vi "Case Structure Test.vi"() -> ()   [LabVIEW 2019]
uses:
  <vilib>/gpm_packages/@cs/test-executive/Source/Test Executive/TestExecutive/Test Executive.lvclass
  C:/Program Files/National Instruments/LabVIEW 2019/vi.lib/gpm_packages/@cs/test-executive/Source/Test Executive/ITestExecutive/ITest Executive.lvclass
  <vilib>/gpm_packages/@cs/run-time-assertions/Source/Assert Equal/Assert Equal.lvclass
  C:/Program Files/National Instruments/LabVIEW 2019/vi.lib/gpm_packages/@cs/run-time-assertions/Source/Assert/Assert.lvclass
  <vilib>/gpm_packages/@cs/run-time-assertions/Source/Assert Greater/Assert Greater.lvclass
  <vilib>/gpm_packages/@cs/run-time-assertions/Source/Assert Less/Assert Less.lvclass
  <vilib>/gpm_packages/@cs/test-executive/Source/Test Executive/Executioner/Executioner.lvclass
  <vilib>/gpm_packages/@cs/persistence/source/XML/XML.lvclass
  C:/Program Files/National Instruments/LabVIEW 2019/vi.lib/gpm_packages/@cs/persistence/source/IPersist/IPersist.lvclass
  e472b746-f4c1-47e9-9711-c7fa7be09181.vi
  ab0fdcf2-3a2d-4a0b-9adf-5da32de36cdd.vi
  99c89cbf-b02e-47c8-8025-58ec5524d82c.vi
  fd6ea1e6-9cba-4bab-b7d6-62b422661ca4.vi
  21af0a36-f5b0-40a4-aa97-dd1ed5091c43.vi
  9cf53736-387a-4554-ab29-2a757f105b86.vi
  bc4700c4-b3ec-42c3-ab81-83467d48079d.vi
  <vilib>/Utility/error.llb/Error Cluster From Error Code.vi
  <vilib>/gpm_packages/@cs/test-executive/Source/Test Executive/ITestExecutive/ITest Executive.lvclass
  <vilib>/gpm_packages/@cs/test-executive/Source/Test Executive/TestExecutive Ref/TestExecutive Ref.lvclass
panel:
  out "Conditional Branches In":string[](array[string])
  out "Conditional Branches out":string[](array[string])
  in  "stop 2":bool
  in  "stop":bool
  in  "Tree":string(tree)
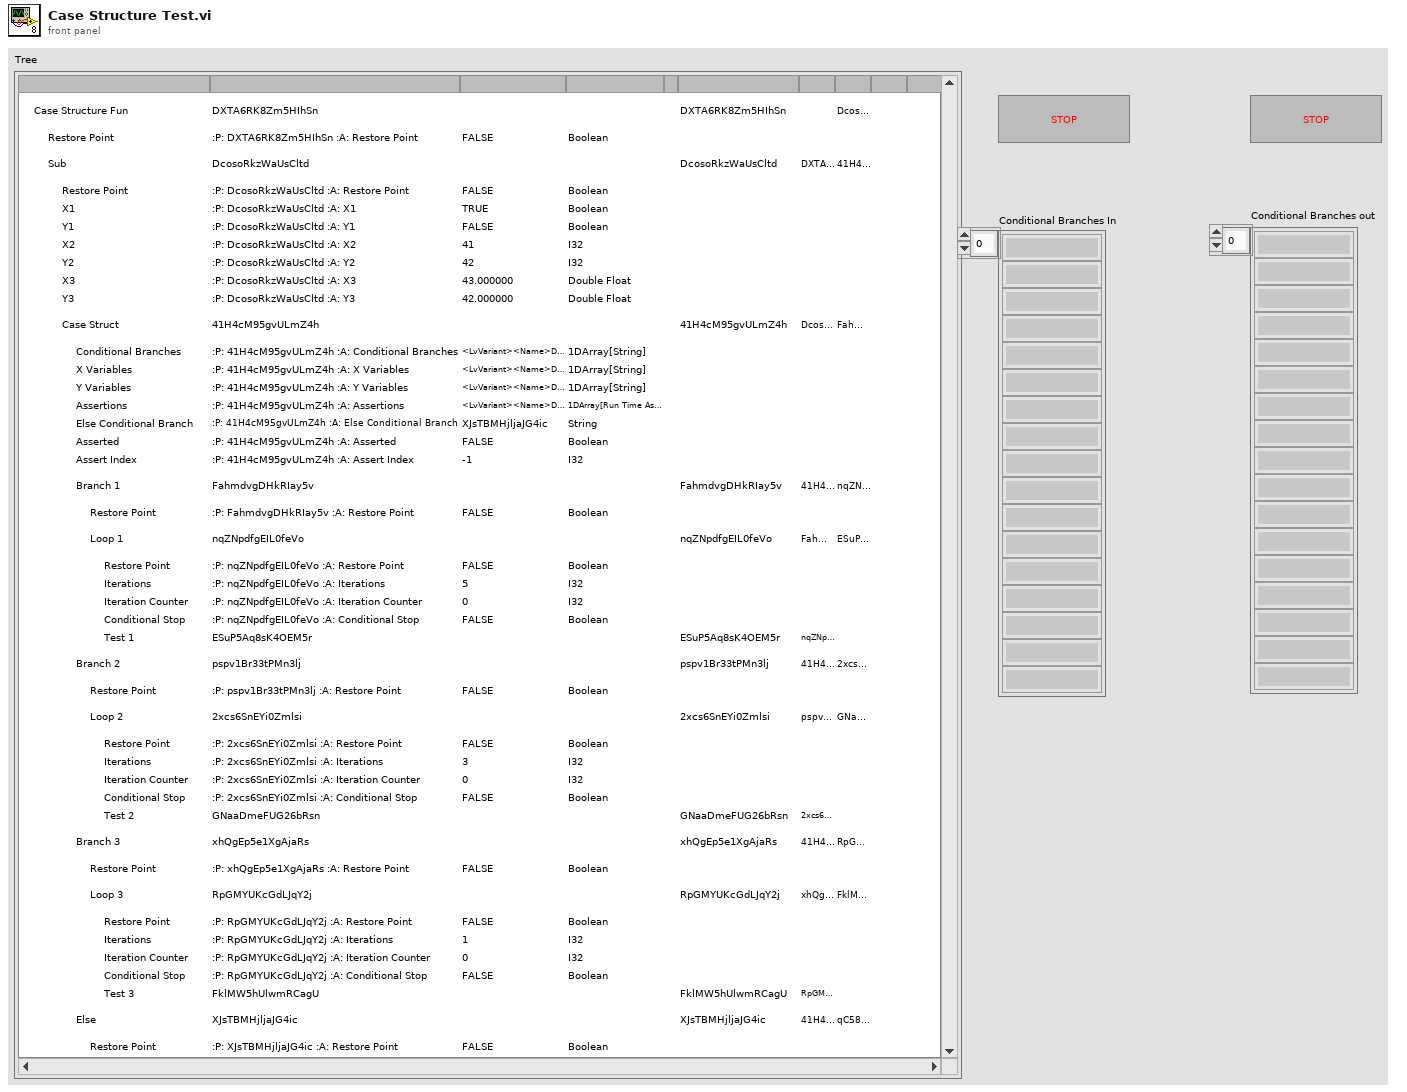
[diagram p1: front panel]
types:
  T1 = cluster{"Left Cell String":string, "Child Text":string[], "Child Tag":string, "Item Indent":i32, "Child Only?":bool, "Glyph Index":i32}[]
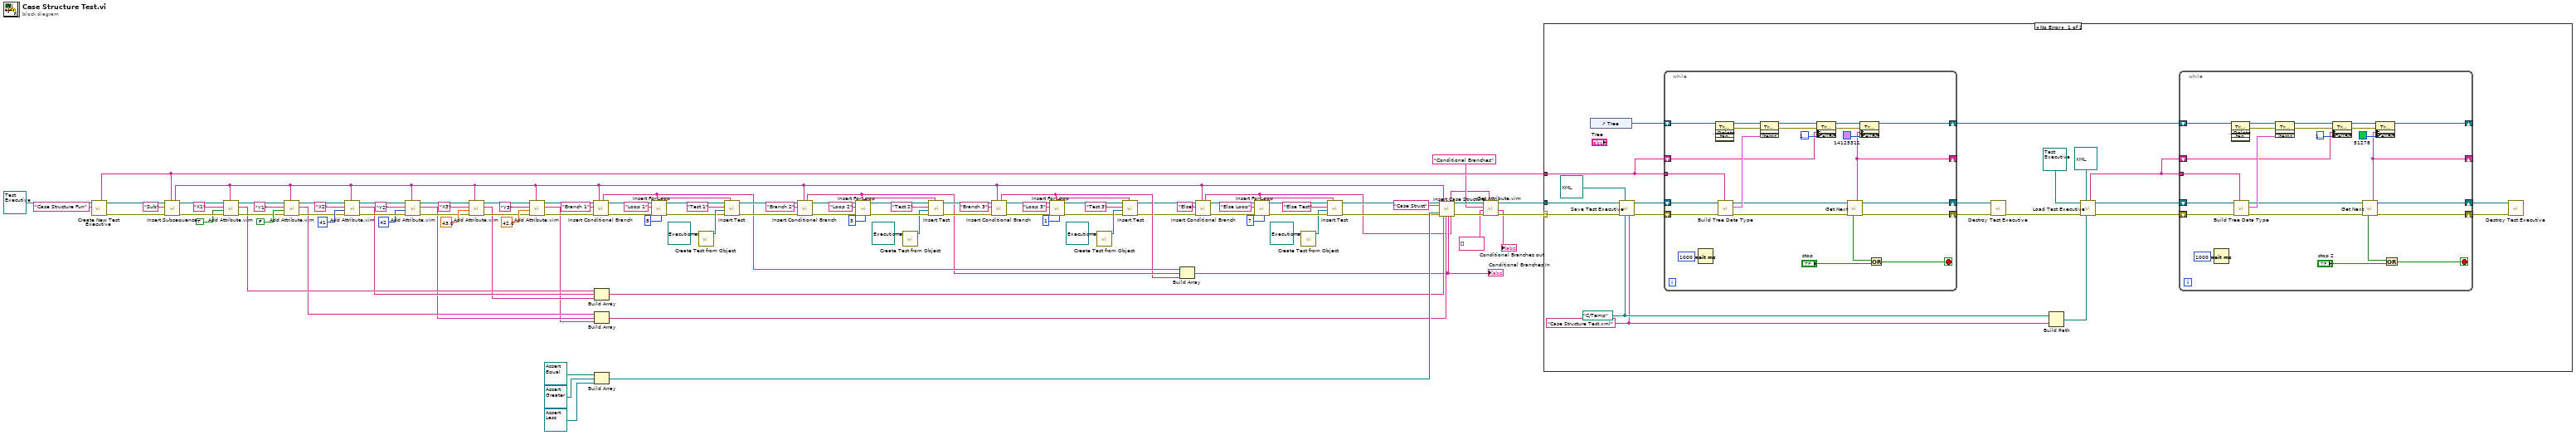
[diagram p0: block diagram]
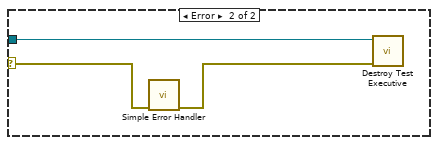
[diagram p2: hidden frame]
diagram:
  n1 = call <vilib>:"Create New Test Executive.vi"("Name"="Case Structure Fun", "Test Executive"=refnum<class "Test Executive.lvclass"> refnum ("Test Executive.lvlib:Test Executive.lvclass")) -> ("error out"=w107:errorcluster, "Test Executive Ref"=w109:refnum<data-value>, "Test Executive ID out"=w11:string)  [unwired: 7 in]
  n2 = call <vilib>:"Insert Subsequence.vi"("Parent ID"=w11, "error in (no error)"=w107, "Name"="Sub", "Test Executive Ref"=w109) -> ("error out"=w105:errorcluster, "Test Executive Ref out"=w106:refnum<data-value>, "Unique ID out"=w7:string)  [unwired: 4 in, 1 out]
  n3 = call "Add Attribute.vim"("ID"=w7, "error in (no error)"=w105, "Attribute"=TRUE, "Attribute Name"="X1", "Test Executive Ref"=w106) -> ("error out"=w99:errorcluster, "Attribute ID out"=w39:string, "Test Executive Ref out"=w100:refnum<data-value>)  [unwired: 3 in, 1 out]
  n4 = call "Add Attribute.vim"("ID"=w7, "error in (no error)"=w99, "Attribute"=FALSE, "Attribute Name"="Y1", "Test Executive Ref"=w100) -> ("error out"=w91:errorcluster, "Attribute ID out"=w36:string, "Test Executive Ref out"=w92:refnum<data-value>)  [unwired: 3 in, 1 out]
  n5 = call "Add Attribute.vim"("ID"=w7, "error in (no error)"=w91, "Attribute"=41, "Attribute Name"="X2", "Test Executive Ref"=w92) -> ("error out"=w98:errorcluster, "Attribute ID out"=w38:string, "Test Executive Ref out"=w97:refnum<data-value>)  [unwired: 3 in, 1 out]
  n6 = call "Add Attribute.vim"("ID"=w7, "error in (no error)"=w98, "Attribute"=42, "Attribute Name"="Y2", "Test Executive Ref"=w97) -> ("error out"=w83:errorcluster, "Attribute ID out"=w35:string, "Test Executive Ref out"=w84:refnum<data-value>)  [unwired: 3 in, 1 out]
  n7 = call "Add Attribute.vim"("ID"=w7, "error in (no error)"=w83, "Attribute"=43.0, "Attribute Name"="X3", "Test Executive Ref"=w84) -> ("error out"=w85:errorcluster, "Attribute ID out"=w37:string, "Test Executive Ref out"=w86:refnum<data-value>)  [unwired: 3 in, 1 out]
  n8 = call "Add Attribute.vim"("ID"=w7, "error in (no error)"=w85, "Attribute"=42.0, "Attribute Name"="Y3", "Test Executive Ref"=w86) -> ("error out"=w80:errorcluster, "Attribute ID out"=w34:string, "Test Executive Ref out"=w82:refnum<data-value>)  [unwired: 3 in, 1 out]
  n9 = call <vilib>:"Insert Conditional Branch.vi"("Parent ID"=w7, "error in (no error)"=w80, "Name"="Branch 1", "Test Executive Ref"=w82) -> ("error out"=w76:errorcluster, "Test Executive Ref out"=w78:refnum<data-value>, "Unique ID out"=w31:string)  [unwired: 4 in, 1 out]
  n10 = Build Array(w39, w38, w37) -> (w33:string[])
  n11 = Build Array(w36, w35, w34) -> (w32:string[])
  n12 = Build Array(refnum<class "Assert Equal.lvclass"> refnum ("Run Time Assertions.lvlib:Assert Equal.lvclass"), refnum<class "Assert Greater.lvclass"> refnum ("Run Time Assertions.lvlib:Assert Greater.lvclass"), refnum<class "Assert Less.lvclass"> refnum ("Run Time Assertions.lvlib:Assert Less.lvclass")) -> (w40:refnum<class "Assert.lvclass">[])
  n13 = call <vilib>:"Insert For Loop.vi"("Loop Iterations"=5, "Parent ID"=w31, "error in (no error)"=w76, "Name"="Loop 1", "Test Executive Ref"=w78) -> ("error out"=w72:errorcluster, "Test Executive Ref out"=w71:refnum<data-value>, "Unique ID out"=w70:string)  [unwired: 3 in, 1 out]
  n14 = call <vilib>:"Create Test from Object.vi"("Test"=refnum<class "Executioner.lvclass"> refnum ("Test Executive.lvlib:Executioner.lvclass")) -> ("Test"=w73:refnum<class "Executioner.lvclass">)  [unwired: 10 in]
  n15 = call <vilib>:"Insert Test.vi"("Parent ID"=w70, "error in (no error)"=w72, "Test"=w73, "Name"="Test 1", "Test Executive Ref"=w71) -> ("error out"=w57:errorcluster, "Test Executive Ref out"=w58:refnum<data-value>)  [unwired: 3 in, 2 out]
  n16 = call <vilib>:"Insert Conditional Branch.vi"("Parent ID"=w7, "error in (no error)"=w57, "Name"="Branch 2", "Test Executive Ref"=w58) -> ("error out"=w63:errorcluster, "Test Executive Ref out"=w61:refnum<data-value>, "Unique ID out"=w30:string)  [unwired: 4 in, 1 out]
  n17 = call <vilib>:"Insert For Loop.vi"("Loop Iterations"=3, "Parent ID"=w30, "error in (no error)"=w63, "Name"="Loop 2", "Test Executive Ref"=w61) -> ("error out"=w67:errorcluster, "Test Executive Ref out"=w68:refnum<data-value>, "Unique ID out"=w69:string)  [unwired: 3 in, 1 out]
  n18 = call <vilib>:"Create Test from Object.vi"("Test"=refnum<class "Executioner.lvclass"> refnum ("Test Executive.lvlib:Executioner.lvclass")) -> ("Test"=w66:refnum<class "Executioner.lvclass">)  [unwired: 10 in]
  n19 = call <vilib>:"Insert Test.vi"("Parent ID"=w69, "error in (no error)"=w67, "Test"=w66, "Name"="Test 2", "Test Executive Ref"=w68) -> ("error out"=w44:errorcluster, "Test Executive Ref out"=w45:refnum<data-value>)  [unwired: 3 in, 2 out]
  n20 = call <vilib>:"Insert Conditional Branch.vi"("Parent ID"=w7, "error in (no error)"=w44, "Name"="Branch 3", "Test Executive Ref"=w45) -> ("error out"=w52:errorcluster, "Test Executive Ref out"=w54:refnum<data-value>, "Unique ID out"=w29:string)  [unwired: 4 in, 1 out]
  n21 = call <vilib>:"Insert For Loop.vi"("Loop Iterations"=1, "Parent ID"=w29, "error in (no error)"=w52, "Name"="Loop 3", "Test Executive Ref"=w54) -> ("error out"=w48:errorcluster, "Test Executive Ref out"=w47:refnum<data-value>, "Unique ID out"=w46:string)  [unwired: 3 in, 1 out]
  n22 = call <vilib>:"Create Test from Object.vi"("Test"=refnum<class "Executioner.lvclass"> refnum ("Test Executive.lvlib:Executioner.lvclass")) -> ("Test"=w49:refnum<class "Executioner.lvclass">)  [unwired: 10 in]
  n23 = call <vilib>:"Insert Test.vi"("Parent ID"=w46, "error in (no error)"=w48, "Test"=w49, "Name"="Test 3", "Test Executive Ref"=w47) -> ("error out"=w15:errorcluster, "Test Executive Ref out"=w16:refnum<data-value>)  [unwired: 3 in, 2 out]
  n24 = Build Array(w31, w30, w29) -> (w28:string[])
  "Conditional Branches In" <- w28
  n25 = call <vilib>:"Insert Conditional Branch.vi"("Parent ID"=w7, "error in (no error)"=w15, "Name"="Else", "Test Executive Ref"=w16) -> ("error out"=w21:errorcluster, "Test Executive Ref out"=w19:refnum<data-value>, "Unique ID out"=w12:string)  [unwired: 4 in, 1 out]
  n26 = call <vilib>:"Insert For Loop.vi"("Loop Iterations"=7, "Parent ID"=w12, "error in (no error)"=w21, "Name"="Else Loop", "Test Executive Ref"=w19) -> ("error out"=w25:errorcluster, "Test Executive Ref out"=w26:refnum<data-value>, "Unique ID out"=w27:string)  [unwired: 3 in, 1 out]
  n27 = call <vilib>:"Create Test from Object.vi"("Test"=refnum<class "Executioner.lvclass"> refnum ("Test Executive.lvlib:Executioner.lvclass")) -> ("Test"=w24:refnum<class "Executioner.lvclass">)  [unwired: 10 in]
  n28 = call <vilib>:"Insert Test.vi"("Parent ID"=w27, "error in (no error)"=w25, "Test"=w24, "Name"="Else Test", "Test Executive Ref"=w26) -> ("error out"=w14:errorcluster, "Test Executive Ref out"=w13:refnum<data-value>)  [unwired: 3 in, 2 out]
  n29 = call <vilib>:"Insert Case Structure.vi"("Test Executive Ref"=w13, "Name"="Case Struct", "Assertions"=w40, "error in (no error)"=w14, "Parent ID"=w7, "X Variables"=w33, "Y Variables"=w32, "Conditional Branches"=w28, "\"Else\" Conditional Branch"=w12) -> ("Unique ID out"=w1:string, "Test Executive Ref out"=w9:refnum<data-value>, "error out"=w6:errorcluster)  [unwired: 7 in, 1 out]
  n30 = call "Get Attribute.vim"("ID"=w1, "error in (no error)"=w6, "Type"=string[] [], "Attribute Name"="Conditional Branches", "Test Executive Ref"=w9) -> ("error out"=w5:errorcluster, "Attribute"=→"Conditional Branches out":string[], "Test Executive Ref out"=w8:refnum<data-value>)  [unwired: 2 in, 2 out]
  n31 = case shown="No Error" w5 {
    selector: w5 -> [w126 w182]
    tunnel: w11 -> [w129 _]
    tunnel: w8 -> [w128 w183]
    frame No Error {
      w118 = "Case Structure Test.xml" ("File Name")
      w119 = path "C:/Temp" ("Folder")
      n32 = control-ref of="Tree"() -> (w132:refnum<vi>)
      n33 = call <vilib>:"Save Test Executive.vi"("File Name"=w118, "Folder"=w119, "Persistence in"=refnum<class "XML.lvclass"> refnum ("XML.lvlib:XML.lvclass"), "error in (no error)"=w126, "Test Executive Ref"=w128) -> ("error out"=w125:errorcluster, "Test Executive Ref out"=w127:refnum<data-value>)  [unwired: 5 in]
      n34 = while {
        tunnel: w129 -> [w163]
        shift-right: [w173] -> w131
        shift-left: w127 -> [w180]
        shift-right: [w171] -> w130
        shift-left: w125 -> [w179]
        shift-right: [w161] -> _
        shift-left: w129 -> [w162]
        shift-right: [w157] -> w115
        shift-left: w132 -> [w177]
        stop <- w158 stop-if-true
        n35 = Wait (ms)(milliseconds to wait=u32 1000) -> ()  [unwired: 1 out]
        n36 = invoke on="Invoke Node" class="Tree (strict)" method="Edit Tree Items.Delete"(reference=w177) -> (reference out=w176:refnum<vi>, error out=w178:errorcluster)  [unwired: 4 in, 3 out]
        n37 = call <vilib>:"Build Tree Data Type.vi"("Test ID"=w163, "error in (no error)"=w179, "Test Executive Ref"=w180) -> ("error out"=w172:errorcluster, "Tree Data"=w175:T1, "Test Executive Ref out"=w174:refnum<data-value>)  [unwired: 6 in]
        n38 = invoke on="Invoke Node" class="Tree (strict)" method="Edit Tree Items.Add Multiple Items to End"(reference=w176, error in=w178, "Items"=w175) -> (reference out=w166:refnum<vi>, error out=w165:errorcluster)  [unwired: 1 in, 2 out]
        n39 = property on="Property Node" class="Tree (strict)"(reference=w166, error in=w165, "Active Item Tag"=w162, "CellBG"=u32 16777226) -> (reference out=w168:refnum<vi>, error out=w164:errorcluster)
        n40 = call <vilib>:"Get Next.vi"("error in (no error)"=w172, "Test Executive Ref"=w174) -> ("error out"=w171:errorcluster, "Test Executive Ref out"=w173:refnum<data-value>, "Unique ID out"=w161:string, "Complete"=w160:bool)  [unwired: 3 in, 3 out]
        n41 = property on="Property Node" class="Tree (strict)"(reference=w168, error in=w164, "Active Item Tag"=w161, "CellBG"=u32 14125311) -> (reference out=w157:refnum<vi>)  [unwired: 1 out]
        n42 = Or(x=w160, y="stop") -> (x .or. y?=w158:bool)
      }
      n43 = call <vilib>:"Destroy Test Executive.vi"("error in (no error)"=w130, "Test Executive Ref"=w131) -> ("error out"=w123:errorcluster)  [unwired: 9 in]
      n44 = Build Path(base path=w119, name or relative path=w118) -> (appended path=w120:path)
      n45 = call <vilib>:"Load Test Executive.vi"("Folder"=w120, "Persistence in"=refnum<class "XML.lvclass"> refnum ("XML.lvlib:XML.lvclass"), "error in (no error)"=w123, "Test Executive"=refnum<class "Test Executive.lvclass"> refnum ("Test Executive.lvlib:Test Executive.lvclass")) -> ("error out"=w116:errorcluster, "Test Executive Ref out"=w117:refnum<data-value>, "Root ID"=w114:string)  [unwired: 5 in]
      n46 = while {
        tunnel: w114 -> [w139]
        shift-right: [w149] -> w113
        shift-left: w117 -> [w156]
        shift-right: [w147] -> w112
        shift-left: w116 -> [w155]
        shift-right: [w137] -> _
        shift-left: w114 -> [w138]
        shift-right: [w133] -> _
        shift-left: w115 -> [w153]
        stop <- w134 stop-if-true
        n47 = Wait (ms)(milliseconds to wait=u32 1000) -> ()  [unwired: 1 out]
        n48 = invoke on="Invoke Node" class="Tree (strict)" method="Edit Tree Items.Delete"(reference=w153) -> (reference out=w152:refnum<vi>, error out=w154:errorcluster)  [unwired: 4 in, 3 out]
        n49 = call <vilib>:"Build Tree Data Type.vi"("Test ID"=w139, "error in (no error)"=w155, "Test Executive Ref"=w156) -> ("error out"=w148:errorcluster, "Tree Data"=w151:T1, "Test Executive Ref out"=w150:refnum<data-value>)  [unwired: 6 in]
        n50 = invoke on="Invoke Node" class="Tree (strict)" method="Edit Tree Items.Add Multiple Items to End"(reference=w152, error in=w154, "Items"=w151) -> (reference out=w142:refnum<vi>, error out=w141:errorcluster)  [unwired: 1 in, 2 out]
        n51 = property on="Property Node" class="Tree (strict)"(reference=w142, error in=w141, "Active Item Tag"=w138, "CellBG"=u32 16777226) -> (reference out=w144:refnum<vi>, error out=w140:errorcluster)
        n52 = call <vilib>:"Get Next.vi"("error in (no error)"=w148, "Test Executive Ref"=w150) -> ("error out"=w147:errorcluster, "Test Executive Ref out"=w149:refnum<data-value>, "Unique ID out"=w137:string, "Complete"=w136:bool)  [unwired: 3 in, 3 out]
        n53 = property on="Property Node" class="Tree (strict)"(reference=w144, error in=w140, "Active Item Tag"=w137, "CellBG"=u32 51278) -> (reference out=w133:refnum<vi>)  [unwired: 1 out]
        n54 = Or(x=w136, y="stop 2") -> (x .or. y?=w134:bool)
      }
      n55 = call <vilib>:"Destroy Test Executive.vi"("error in (no error)"=w112, "Test Executive Ref"=w113) -> ()  [unwired: 9 in, 1 out]
    }
    frame Error {
      n56 = call <vilib>:"Simple Error Handler.vi"("error in (no error)"=w182) -> ("error out"=w181:errorcluster)  [unwired: 4 in, 4 out]
      n57 = call <vilib>:"Destroy Test Executive.vi"("error in (no error)"=w181, "Test Executive Ref"=w183) -> ()  [unwired: 9 in, 1 out]
    }
  }
